vi "iteration_timer.vi"() -> ()   [LabVIEW 2020]
panel:
  out "Waveform Chart":dbl[](graph)
  out "deltat":dbl
  in  "stop":bool
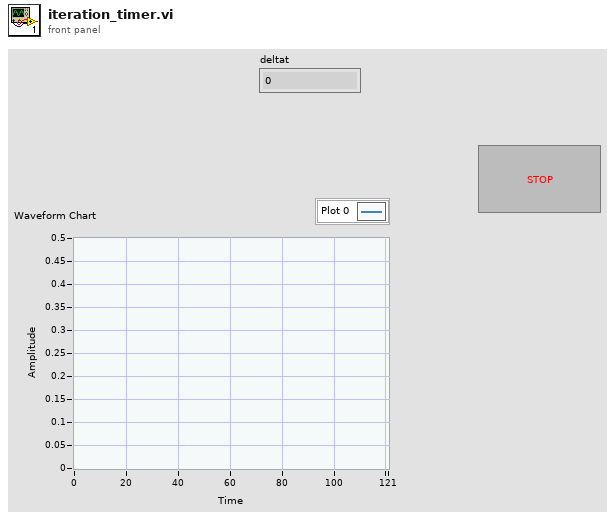
[diagram p1: front panel]
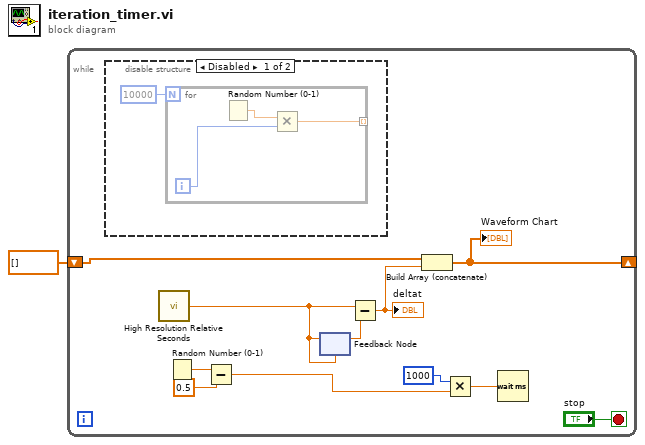
[diagram p0: block diagram]
diagram:
  n1 = while {
    shift-right: [w7] -> _
    shift-left: dbl[] [] -> [w8]
    stop <- "stop" stop-if-true
    n2 = disable-structure shown="Disabled" {
      frame Disabled {
        n3 = for {
          N: 10000 -> [_]
          tunnel: [w14] -> _ mode=indexing
          i -> [w15]
          n4 = Random Number (0-1)() -> (number: 0 to 1=w16:dbl)
          n5 = Multiply(x=w16, y=w15) -> (x*y=w14:dbl)
        }
      }
      frame Enabled {
      }
    }
    n6 = call <vilib>:"High Resolution Relative Seconds.vi"() -> ("relative seconds"=w10:dbl)
    n7 = Random Number (0-1)() -> (number: 0 to 1=w6:dbl)
    n8 = Subtract(x=w6, y=0.5) -> (x-y=w3:dbl)
    n9 = feedback-in #1(w10) -> ()
    n10 = feedback #1(w10) -> (w11:dbl)
    n11 = Subtract(x=w10, y=w11) -> (x-y=w9:dbl)
    "deltat" <- w9
    n12 = Build Array (concatenate)(w8, w9) -> (w7:dbl[])
    "Waveform Chart" <- w7
    n13 = Multiply(x=u32 1000 ("milliseconds to wait"), y=w3) -> (x*y=w2:dbl)
    n14 = Wait (ms)(milliseconds to wait=w2) -> ()  [unwired: 1 out]
  }
